vi "Invert Colour.vi"(8 "error in (no error)":errorcluster, 11 "Colour":u32(colorbox)) -> (0 "error out":errorcluster, 3 "Inverted Colour":u32(colorbox)=16777215)   [LabVIEW 2018, in "Colour Lab.lvlib"]
uses:
  Colour Lab.lvlib
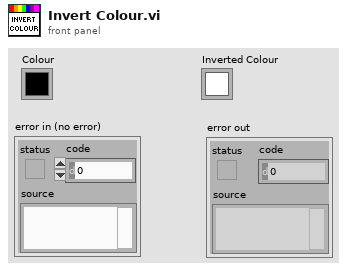
[diagram p1: front panel]
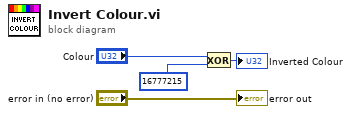
[diagram p0: block diagram]
diagram:
  n1 = Exclusive Or(1:u32 16777215, 2:"Colour") -> (0:→"Inverted Colour":u32)
  "error out" <- "error in (no error)"
